vi "detDirWall.vi"(1 "Radius":i32, 2 "Y-cord":i32, 3 "X-cord":i32, 4 "Source Image":T1(plugin-control)) -> (0 "Angle dir":i32)   [LabVIEW 2009, in "ImageAnalysis.lvlib"]
uses:
  ImageAnalysis.lvlib
  <vilib>/vision/NI_Vision_Development_Module.lvlib
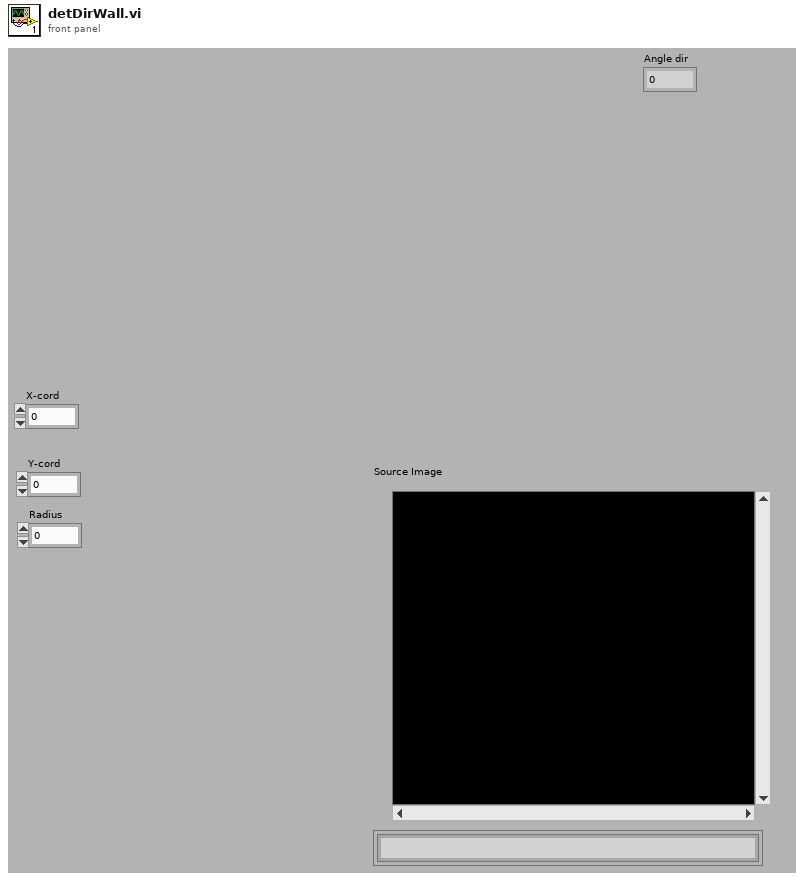
[diagram p1: front panel]
types:
  T1 = typedef "IMAQ Image.ctl" = refnum<image>
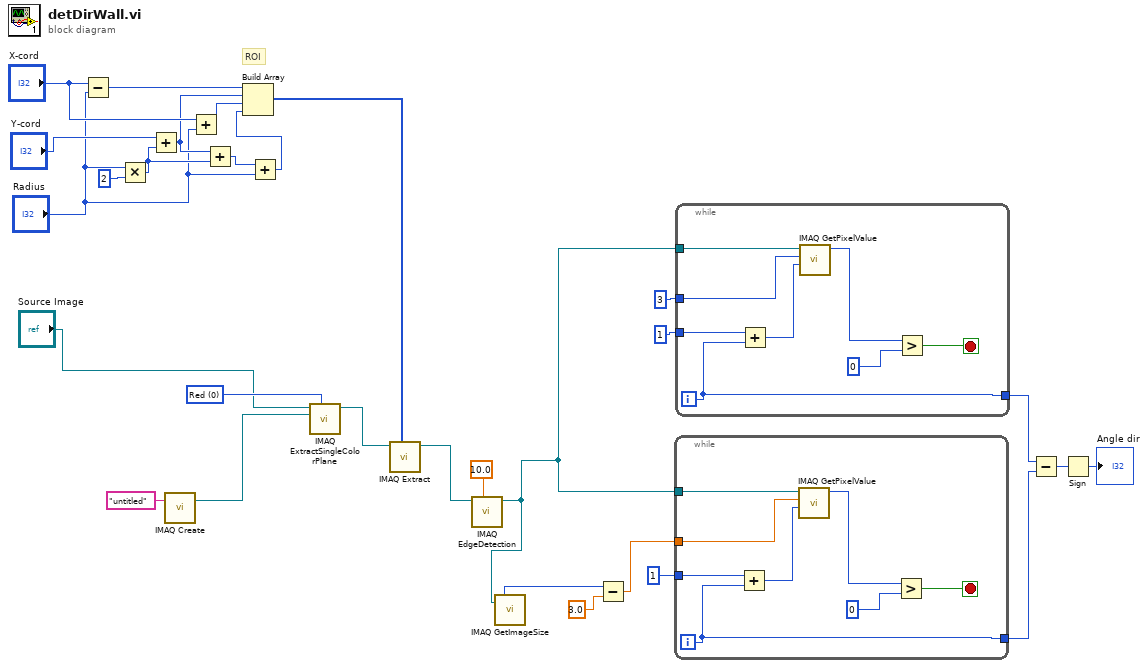
[diagram p0: block diagram]
diagram:
  w29 = 0 items=["Red", "Green", "Blue", "Hue", "Saturation", "Luminance", "Value", "Intensity"] ("Color Plane")
  # "ROI"
  n1 = Subtract(x="X-cord", y="Radius") -> (x-y=w16:i32)
  n2 = Multiply(x="Radius", y=2) -> (x*y=w10:i32)
  n3 = Add(x="Y-cord", y=w10) -> (x+y=w11:i32)
  n4 = call "IMAQ Create"("Image Name"="untitled") -> ("New Image"=w5:T1)  [unwired: 4 in, 1 out]
  n5 = Add(x="X-cord", y="Radius") -> (x+y=w15:i32)
  n6 = Add(x=w11, y=w10) -> (x+y=w8:i32)
  n7 = Add(x=w8, y="Radius") -> (x+y=w7:i32)
  n8 = Build Array(w16, w11, w15, w7) -> (w3:i32[])
  n9 = call "IMAQ ExtractSingleColorPlane"("Color Plane"=w29, "Image Dst"=w5, "Image Src"="Source Image") -> ("Image Dst Out"=w1:T1)  [unwired: 7 in, 1 out]
  n10 = call "IMAQ Extract"("Optional Rectangle"=w3, "Image Src"=w1) -> ("Image Dst Out"=w2:T1)  [unwired: 8 in, 1 out]
  n11 = call "IMAQ EdgeDetection"("Threshold Value"=sgl 10.0, "Image Src"=w2) -> ("Image Dst Out"=w20:T1)  [unwired: 8 in, 1 out]
  n12 = call "IMAQ GetImageSize"("Image"=w20) -> ("X Resolution"=w18:i32)  [unwired: 3 in, 2 out]
  n13 = Subtract(x=w18, y=3.0) -> (x-y=w17:dbl)
  n14 = while {
    tunnel: w20 -> [w37]
    tunnel: [w33] -> w23
    tunnel: w17 -> [w32]
    tunnel: 1 ("Y Coordinate") -> [w31]
    i -> [w33]
    stop <- w34 stop-if-true
    n15 = Add(x=w31, y=w33) -> (x+y=w30:i32)
    n16 = call "IMAQ GetPixelValue"("Image"=w37, "X Coordinate"=w32, "Y Coordinate"=w30) -> ("Pixel Value (U8)"=w36:u8)  [unwired: 3 in, 4 out]
    n17 = Greater?(x=w36, y=u8 0) -> (0:w34:bool)
  }
  n18 = while {
    tunnel: w20 -> [w45]
    tunnel: [w41] -> w24
    tunnel: 3 ("X Coordinate") -> [w40]
    tunnel: 1 ("Y Coordinate") -> [w39]
    i -> [w41]
    stop <- w42 stop-if-true
    n19 = Add(x=w39, y=w41) -> (x+y=w38:i32)
    n20 = call "IMAQ GetPixelValue"("Image"=w45, "X Coordinate"=w40, "Y Coordinate"=w38) -> ("Pixel Value (U8)"=w44:u8)  [unwired: 3 in, 4 out]
    n21 = Greater?(x=w44, y=u8 0) -> (0:w42:bool)
  }
  n22 = Subtract(x=w24, y=w23) -> (x-y=w21:i32)
  n23 = Sign(1:w21) -> (0:→"Angle dir":i32)
